vi "Rename TDMS Property.vi"() -> ()   [LabVIEW 2011]
uses:
  server/database/Fields/Field DataTypes.ctl
  Summitek EXT/OpenG EXT/file/file.llb/File Exists - Scalar__ogtk.vi
  Summitek EXT/OpenG EXT/file/file.llb/Strip Path Extension - String__ogtk.vi
panel:
  in  "Units":string
  in  "Data Type":T1
  in  "Run Number (-1 = Latest, -2 = All)":i32=-2
  out "error out":errorcluster
  in  "error in (no error)":errorcluster
  in  "TDMS File or Folder":path
  in  "New Value":string
  in  "sxFieldId":string
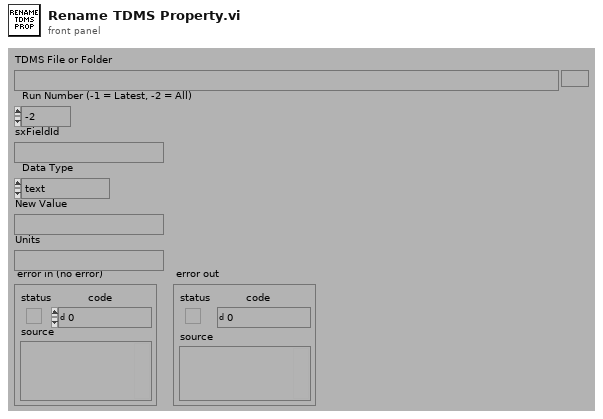
[diagram p1: front panel]
types:
  T1 = typedef "Field DataTypes.ctl" = enum32{"text", "numeric", "list", "timestamp", "boolean"}
  T2 = enum16{"open", "open or create", "create or replace", "create", "open (read-only)"}
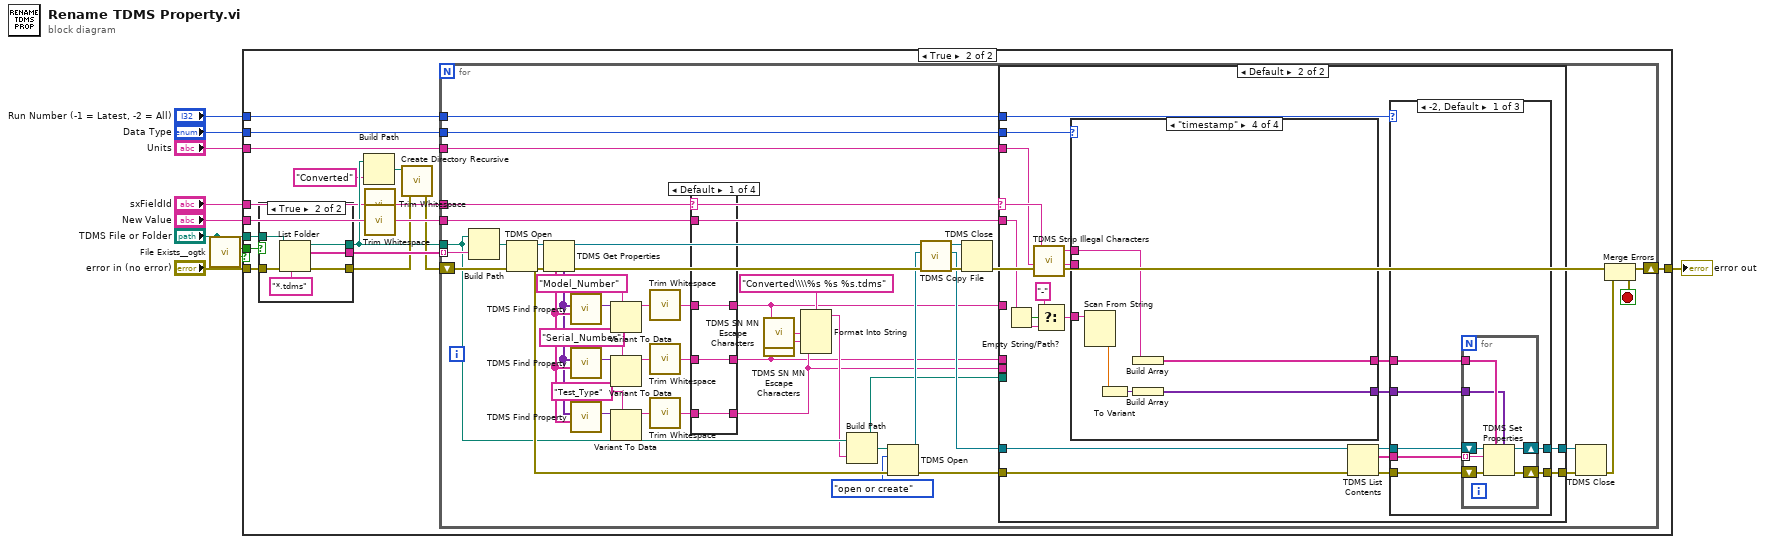
[diagram p0: block diagram]
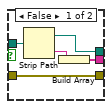
[diagram p3: hidden frame]
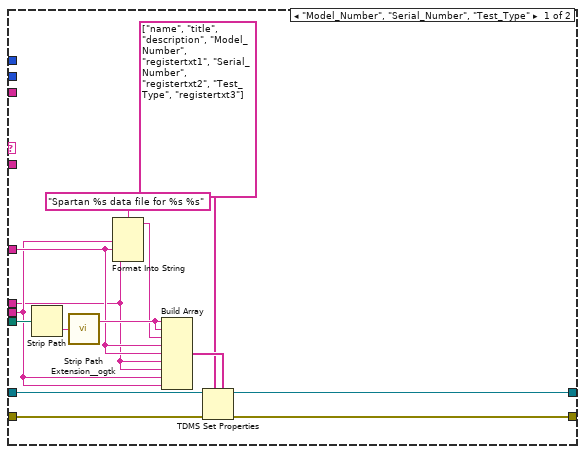
[diagram p7: hidden frame]
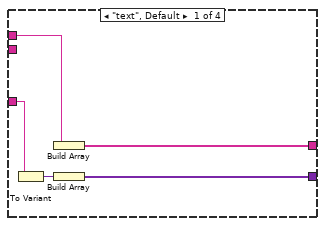
[diagram p8: hidden frame]
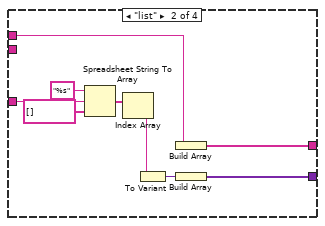
[diagram p9: hidden frame]
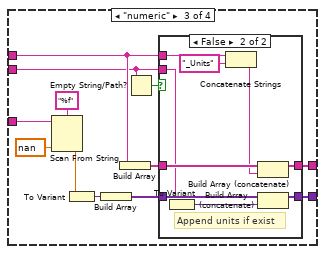
[diagram p10: hidden frame]
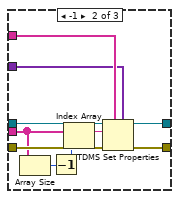
[diagram p12: hidden frame]
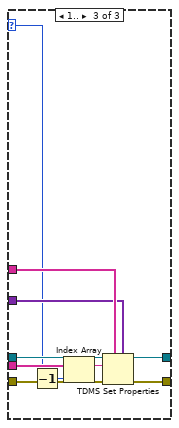
[diagram p13: hidden frame]
diagram:
  n1 = call-poly "File Exists__ogtk.vi"("file path"="TDMS File or Folder") -> ("is directory"=w9:bool, "exists"=w10:bool)  [unwired: 6 in]
  n2 = case shown="True" w10 {
    tunnel: w9 -> [_ w22]
    tunnel: "error in (no error)" -> [w11 w27]
    tunnel: [w11 w25] -> w7
    tunnel: "sxFieldId" -> [_ w13]
    tunnel: "New Value" -> [_ w28]
    tunnel: "TDMS File or Folder" -> [_ w26]
    tunnel: "Run Number (-1 = Latest, -2 = All)" -> [_ w17]
    tunnel: "Data Type" -> [_ w16]
    tunnel: "Units" -> [_ w15]
    frame False {
    }
    frame True {
      n3 = case shown="True" w22 {
        tunnel: w27 -> [w33 w39]
        tunnel: w26 -> [w31 w38]
        tunnel: [w33 w36] -> w21
        tunnel: [w29 w35] -> w19
        tunnel: [w32 w34] -> w24
        frame False {
          n4 = Strip Path(path=w31) -> (stripped path=w29:path, name=w30:string)
          n5 = Build Array(w30) -> (w32:string[])
        }
        frame True {
          n6 = List Folder(path=w38, pattern="*.tdms", error in=w39) -> (path out=w35:path, filenames=w34:string[], error out=w36:errorcluster)  [unwired: 1 in, 1 out]
        }
      }
      n7 = Build Path(base path=w19, name or relative path="Converted") -> (appended path=w18:path)
      n8 = call <vilib>:"Trim Whitespace.vi"("string"=w13) -> ("trimmed string"=w12:string)  [unwired: 1 in]
      n9 = call <vilib>:"Trim Whitespace.vi"("string"=w28) -> ("trimmed string"=w23:string)  [unwired: 1 in]
      n10 = call <vilib>:"Create Directory Recursive.vi"("error in (no error)"=w21, "directory"=w18) -> ("error out"=w20:errorcluster)  [unwired: 1 in, 4 out]
      n11 = for {
        shift-right: [w43] -> w25
        shift-left: w20 -> [w85]
        tunnel: w19 -> [w65]
        tunnel: w24 -> [w84] mode=indexing
        tunnel: w12 -> [w53]
        tunnel: w23 -> [w49]
        tunnel: w17 -> [w42]
        tunnel: w16 -> [w41]
        tunnel: w15 -> [w40]
        stop <- w43 stop-if-true
        w76 = "Test_Type" ("Property Name")
        w77 = "Serial_Number" ("Property Name")
        w78 = "Model_Number" ("Property Name")
        n12 = Build Path(base path=w65, name or relative path=w84) -> (appended path=w83:path)
        n13 = TDMS Open(8:w85, 11:w83) -> (0:w67:errorcluster, 3:w68:refnum<k34>)  [unwired: 4 in]
        n14 = TDMS Get Properties(8:w67, 11:w68) -> (0:w64:errorcluster, 3:w63:refnum<k34>, 4:w81:variant[], 6:w82:string[])  [unwired: 4 in, 2 out]
        n15 = call "TDMS Find Property.vi"("Property Name"=w78, "Property Names"=w82, "Property Values"=w81) -> ("Property Value"=w80:variant)  [unwired: 5 out]
        n16 = call "TDMS Find Property.vi"("Property Name"=w77, "Property Names"=w82, "Property Values"=w81) -> ("Property Value"=w79:variant)  [unwired: 5 out]
        n17 = call "TDMS Find Property.vi"("Property Name"=w76, "Property Names"=w82, "Property Values"=w81) -> ("Property Value"=w75:variant)  [unwired: 5 out]
        n18 = Variant To Data(type=w78, Variant=w80) -> (data=w72:string)  [unwired: 1 in, 1 out]
        n19 = Variant To Data(type=w77, Variant=w79) -> (data=w70:string)  [unwired: 1 in, 1 out]
        n20 = Variant To Data(type=w76, Variant=w75) -> (data=w71:string)  [unwired: 1 in, 1 out]
        n21 = call <vilib>:"Trim Whitespace.vi"("string"=w72) -> ("trimmed string"=w50:string)  [unwired: 1 in]
        n22 = call <vilib>:"Trim Whitespace.vi"("string"=w70) -> ("trimmed string"=w51:string)  [unwired: 1 in]
        n23 = call <vilib>:"Trim Whitespace.vi"("string"=w71) -> ("trimmed string"=w52:string)  [unwired: 1 in]
        n24 = case shown="Default" w53 {
          tunnel: w52 -> [w86 w90 w93 _]
          tunnel: w51 -> [w87 w89 _ w96]
          tunnel: w50 -> [w88 _ w94 w97]
          tunnel: w49 -> [_ w91 w92 w95]
          tunnel: [w88 w91 w94 w97] -> w48
          tunnel: [w86 w90 w93 w95] -> w47
          tunnel: [w87 w89 w92 w96] -> w46
          frame Default {
          }
          frame "Model_Number" {
          }
          frame "Serial_Number" {
          }
          frame "Test_Type" {
          }
        }
        n25 = call "TDMS SN MN Escape Characters.vi"("string"=w48) -> ("url-encoded string"=w69:string)
        n26 = call "TDMS SN MN Escape Characters.vi"("string"=w46) -> ("url-encoded string"=w74:string)
        n27 = Format Into String(format string="Converted\\\\%s %s %s.tdms", w69, w74, w47) -> (resulting string=w55:string)  [unwired: 2 in, 1 out]
        n28 = Build Path(base path=w65, name or relative path=w55) -> (appended path=w54:path)
        n29 = TDMS Open(8:w67, 10:T2."open or create" ("operation (0:open)"), 11:w54) -> (0:w58:errorcluster, 3:w62:refnum<k34>)  [unwired: 3 in]
        n30 = call "TDMS Copy File.vi"("error in"=w64, "tdms dest in"=w62, "tdms source in"=w63) -> ("error out"=w60:errorcluster, "tdms dest out"=w59:refnum<k34>, "tdms source out"=w61:refnum<k34>)  [unwired: 6 in]
        n31 = TDMS Close(8:w60, 11:w61) -> (0:w45:errorcluster)  [unwired: 1 out]
        n32 = case shown="Default" w53 {
          selector: w53 -> [_ w117]
          tunnel: w59 -> [w110 w126]
          tunnel: w58 -> [w111 w127]
          tunnel: [w102 w128] -> w57
          tunnel: [w103 w129] -> w56
          tunnel: w49 -> [_ w114]
          tunnel: w54 -> [w107 _]
          tunnel: w48 -> [w100 _]
          tunnel: w46 -> [w98 _]
          tunnel: w47 -> [w99 _]
          tunnel: w42 -> [_ w122]
          tunnel: w41 -> [_ w116]
          tunnel: w40 -> [_ w115]
          frame "Model_Number", "Serial_Number", "Test_Type" {
            n33 = Strip Path(path=w107) -> (name=w106:string)  [unwired: 1 out]
            n34 = call-poly "Strip Path Extension__ogtk.vi"("path"=w106) -> ("root"=w108:string)  [unwired: 1 out]
            n35 = Format Into String(format string="Spartan %s data file for %s %s", w99, w100, w98) -> (resulting string=w105:string)  [unwired: 2 in, 1 out]
            n36 = Build Array(w108, w108, w105, w100, w100, w98, w98, w99, w99) -> (w104:string[])
            n37 = TDMS Set Properties(5:w104, 7:string[] ["name", "title", "description", "Model_Number", "registertxt1", "Serial_Number", "registertxt2", "Test_Type", "registertxt3"], 8:w111, 11:w110) -> (0:w102:errorcluster, 3:w103:refnum<k34>)  [unwired: 2 in, 2 out]
          }
          frame Default {
            n38 = Empty String/Path?(string/path=w114) -> (empty?=w121:bool)
            n39 = call "TDMS Strip Illegal Characters.vi"("String"=w117) -> ("Legal String"=w118:string)  [unwired: 4 out]
            n40 = Select(t="-", s=w121, f=w114) -> (s? t:f=w120:string)
            n41 = case shown="\"timestamp\"" w116 {
              tunnel: w120 -> [w134 w139 w152 w171]
              tunnel: [w130 w140 w147 w170] -> w113
              tunnel: [w133 w143 w148 w169] -> w112
              tunnel: w118 -> [w131 w141 w146 w168]
              tunnel: w115 -> [_ _ w144 _]
              frame "text", Default {
                n42 = To Variant(anything=w134) -> (Variant=w132:variant)
                n43 = Build Array(w131) -> (w133:string[])
                n44 = Build Array(w132) -> (w130:variant[])
              }
              frame "list" {
                n45 = Spreadsheet String To Array(format string="%s" ("delimiter (Tab)"), spreadsheet string=w139, array type (2D Dbl)=string[] []) -> (array=w137:string[])  [unwired: 1 in]
                n46 = Index Array(array=w137) -> (element=w136:string)  [unwired: 1 in]
                n47 = To Variant(anything=w136) -> (Variant=w142:variant)
                n48 = Build Array(w141) -> (w143:string[])
                n49 = Build Array(w142) -> (w140:variant[])
              }
              frame "numeric" {
                n50 = Scan From String(format string="%f", input string=w152, default 1=nan) -> (output 1=w154:dbl)  [unwired: 2 in, 3 out]
                n51 = To Variant(anything=w154) -> (Variant=w155:variant)
                n52 = Build Array(w155) -> (w149:variant[])
                n53 = Build Array(w146) -> (w150:string[])
                n54 = Empty String/Path?(string/path=w144) -> (empty?=w145:bool)
                n55 = case shown="False" w145 {
                  tunnel: w150 -> [w157 w166]
                  tunnel: w149 -> [w156 w165]
                  tunnel: [w157 w164] -> w148
                  tunnel: [w156 w163] -> w147
                  tunnel: w146 -> [_ w161]
                  tunnel: w144 -> [_ w158]
                  frame True {
                  }
                  frame False {
                    # "Append units if exist"
                    n56 = To Variant(anything=w158) -> (Variant=w159:variant)
                    n57 = Concatenate Strings(w161, "_Units") -> (w160:string)
                    n58 = Build Array (concatenate)(w166, w160) -> (w164:string[])
                    n59 = Build Array (concatenate)(w165, w159) -> (w163:variant[])
                  }
                }
              }
              frame "timestamp" {
                n60 = Scan From String(input string=w171) -> (output 1=w172:dbl)  [unwired: 3 in, 4 out]
                n61 = To Variant(anything=w172) -> (Variant=w167:variant)
                n62 = Build Array(w168) -> (w169:string[])
                n63 = Build Array(w167) -> (w170:variant[])
              }
            }
            n64 = TDMS List Contents(4:w127, 7:w126) -> (0:w124:errorcluster, 2:w123:string[], 3:w125:refnum<k34>)  [unwired: 1 in, 1 out]
            n65 = case shown="-2, Default" w122 {
              selector: w122 -> [_ _ w197]
              tunnel: [w176 w194 w204] -> w129
              tunnel: [w175 w193 w203] -> w128
              tunnel: w125 -> [w178 w196 w206]
              tunnel: w124 -> [w177 w195 w205]
              tunnel: w123 -> [w179 w190 w200]
              tunnel: w112 -> [w174 w192 w202]
              tunnel: w113 -> [w173 w191 w201]
              frame -2, Default {
                n66 = for {
                  tunnel: w179 -> [w184] mode=indexing
                  shift-right: [w180] -> w175
                  shift-left: w177 -> [w185]
                  shift-right: [w181] -> w176
                  shift-left: w178 -> [w186]
                  tunnel: w174 -> [w183]
                  tunnel: w173 -> [w182]
                  n67 = TDMS Set Properties(5:w182, 7:w183, 8:w185, 10:w184, 11:w186) -> (0:w180:errorcluster, 3:w181:refnum<k34>)  [unwired: 1 in, 2 out]
                }
              }
              frame -1 {
                n68 = Array Size(array=w190) -> (size(s)=w189:i32)
                n69 = Decrement(x=w189) -> (x-1=w188:i32)
                n70 = Index Array(array=w190, index=w188) -> (element=w187:string)
                n71 = TDMS Set Properties(5:w191, 7:w192, 8:w195, 10:w187, 11:w196) -> (0:w193:errorcluster, 3:w194:refnum<k34>)  [unwired: 1 in, 2 out]
              }
              frame 1.. {
                n72 = Decrement(x=w197) -> (x-1=w199:i32)
                n73 = Index Array(array=w200, index=w199) -> (element=w198:string)
                n74 = TDMS Set Properties(5:w201, 7:w202, 8:w205, 10:w198, 11:w206) -> (0:w203:errorcluster, 3:w204:refnum<k34>)  [unwired: 1 in, 2 out]
              }
            }
          }
        }
        n75 = TDMS Close(8:w57, 11:w56) -> (0:w44:errorcluster)  [unwired: 1 out]
        n76 = Merge Errors(w45, w44) -> (w43:errorcluster)
      }
    }
  }
  "error out" <- w7
